vi "Main.vi"(11 "Module Admin":refnum<class "Delacor_lib_QMH_Module Admin.lvclass">) -> ()   [LabVIEW 2020, in "Logging.lvlib"]
doc: "This template is based off of the Queued Message Handler design pattern and the Queued Message Handler project template that ships with LabVIEW.\n\nThe main difference is that the queue is private to this module and communication between modules is performed via Broadcast and Request events.\n\nRequest events are wrapped in public API methods and are handled in the Event Handling Loop (EHL) of this VI. Any module can register for Broadcast events sent by this module. The EHL generates messages based on user interface actions.\n\nThe Message Handling Loop (MHL) processes messages generated by the EHL, or by other messages. The messages are string values, so new messages can be added easily to the Message Cases case structure in the MHL. Each message cluster can also provide an optional value for Message Data, which is a variant that can be converted to whatever message-specific data is required.\n_____\nBased on Delacor QMH Project Template 6.0.0.89."
uses:
  Logging.lvlib
  <vilib>/Delacor/Delacor QMH/Libraries/Module Admin_class/Delacor_lib_QMH_Module Admin.lvclass
  Module Data--cluster.ctl
  <vilib>/Delacor/Delacor QMH/Libraries/Message Queue_class/Delacor_lib_QMH_Message Queue.lvclass/Delacor_lib_QMH_Message Queue.ctl
  Stop Argument--cluster.ctl
  <vilib>/Delacor/Delacor QMH/Libraries/Module Admin_class/Delacor_lib_QMH_Module Admin.lvclass/Delacor_lib_QMH_Module Admin.ctl
  <vilib>/Utility/miscctls.llb/LVPointTypeDef.ctl
  <vilib>/Delacor/Delacor QMH/Libraries/Message Queue_class/Delacor_lib_QMH_Enqueue Message (Single).vi
  <vilib>/Delacor/Delacor QMH/Libraries/Module Admin_class/Delacor_lib_QMH_Get External Launch.vi
  <vilib>/Utility/error.llb/Error Cluster From Error Code.vi
  <vilib>/ErrorRing/Error Ring.xnode
  <vilib>/Delacor/Delacor QMH/Libraries/Message Queue_class/Delacor_lib_QMH_Message Queue.lvclass
  Acquisition/Acquisition.lvlib
  Settings/Settings.lvlib
panel:
  in  "TDMS FILE":bool
  in  "NAME":string
  out "error out":errorcluster
  out "Status":string
  in  "Simulate MHL Error":bool
  in  "Simulate EHL Error":bool
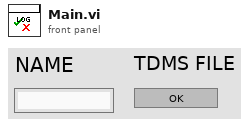
[diagram p1: front panel]
types:
  T1 = typedef "Logging.lvlib/Request Events--cluster.ctl" = cluster{"Stop Module":refnum<user-event>, "Show Panel":refnum<user-event>, "Hide Panel":refnum<user-event>, "Get Module Execution Status":refnum<user-event>, "Show Diagram":refnum<user-event>}
  T2 = typedef "Settings.lvlib/Broadcast Events--cluster.ctl" = cluster{"Module Did Init":refnum<user-event>, "Status Updated":refnum<user-event>, "Error Reported":refnum<user-event>, "Module Did Stop":refnum<user-event>, "Update Module Execution Status":refnum<user-event>, "Task to do":refnum<user-event>, "Nombre task":refnum<user-event>}
  T3 = typedef "Acquisition.lvlib/Broadcast Events--cluster.ctl" = cluster{"Module Did Init":refnum<user-event>, "Status Updated":refnum<user-event>, "Error Reported":refnum<user-event>, "Module Did Stop":refnum<user-event>, "Update Module Execution Status":refnum<user-event>, "Data Analog aquired":refnum<user-event>, "DIGITAL DATA":refnum<user-event>, "TIPO ADQUI":refnum<user-event>}
  T4 = typedef "Logging.lvlib/Module Data--cluster.ctl" = cluster{"Status":string, "ANALOGICO/DIGITAL":bool, "DIGITAL DAQ":bool[], "data":waveform(dbl)[], "NAME":string}
  T5 = enum32{"invalid lock state", "Not Locked", "Locked (No Password)", "Password-protected"}
  T6 = typedef "Logging.lvlib/Stop Argument--cluster.ctl" = cluster{"Origin":string, "Exit via Stop Module Req?":bool, "Wait for Module to stop?":bool}
  T7 = typedef "LVPointTypeDef.ctl" = cluster{"Horizontal":i16, "Vertical":i16}
  T8 = enum32{"Invalid", "Standard", "Closed", "Hidden", "Minimized", "Maximized"}
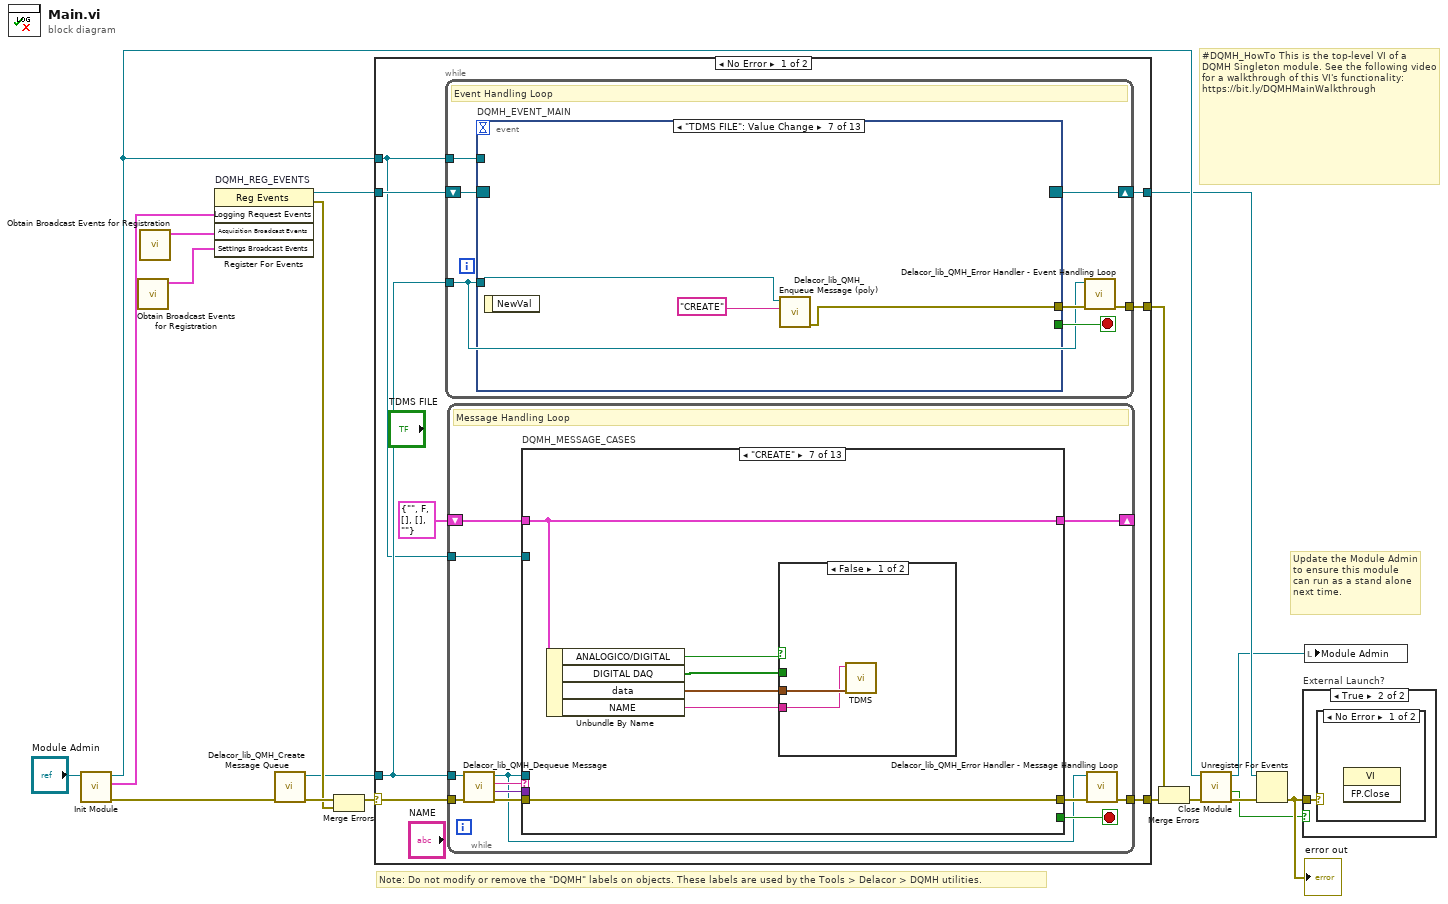
[diagram p0: block diagram]
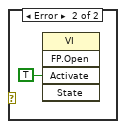
[diagram p3: hidden frame]
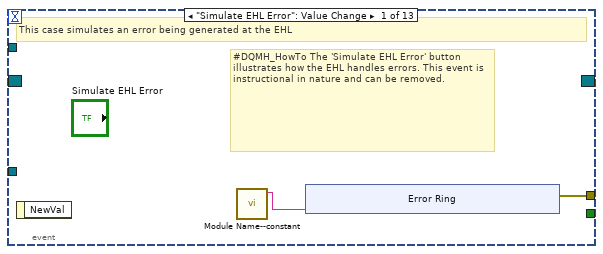
[diagram p4: hidden frame]
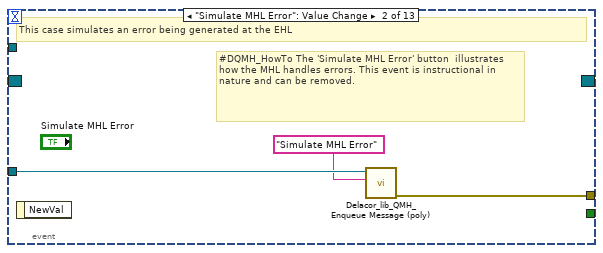
[diagram p5: hidden frame]
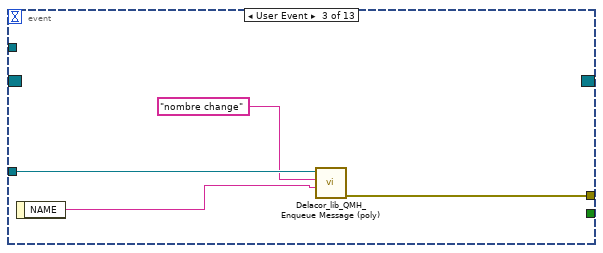
[diagram p6: hidden frame]
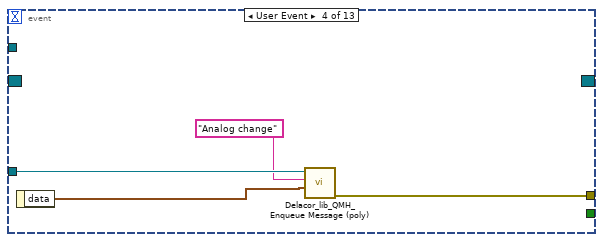
[diagram p7: hidden frame]
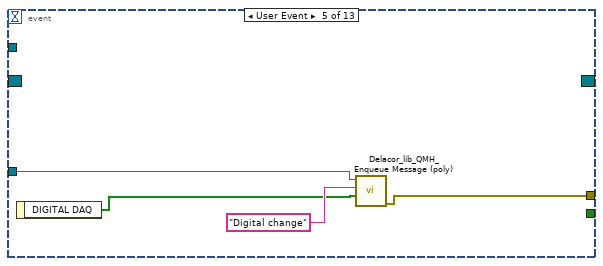
[diagram p8: hidden frame]
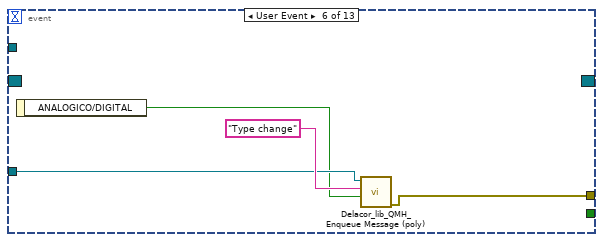
[diagram p9: hidden frame]
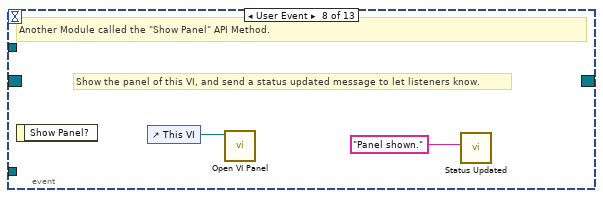
[diagram p10: hidden frame]
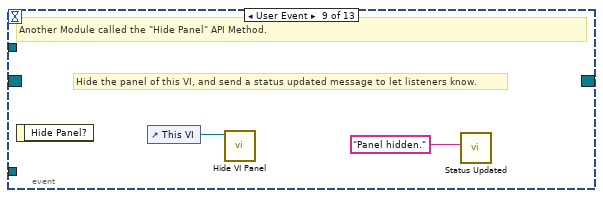
[diagram p11: hidden frame]
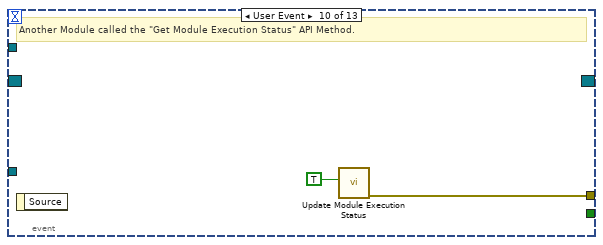
[diagram p12: hidden frame]
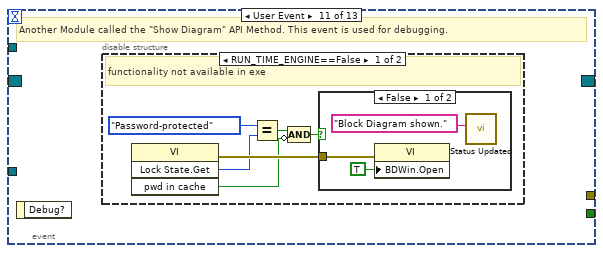
[diagram p13: hidden frame]
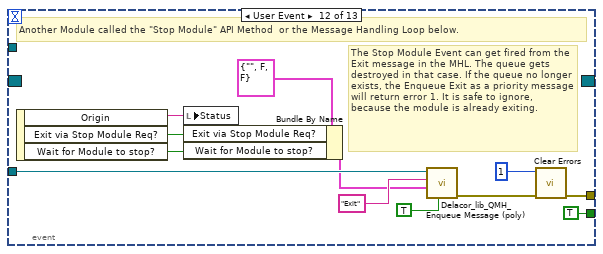
[diagram p16: hidden frame]
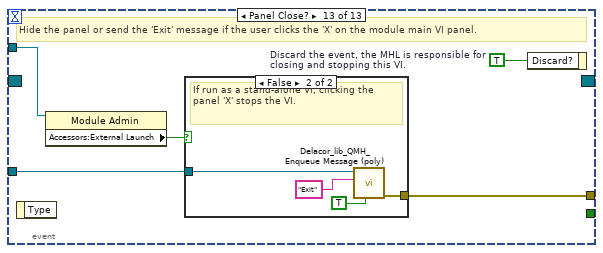
[diagram p17: hidden frame]
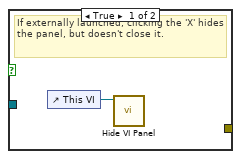
[diagram p18: hidden frame]
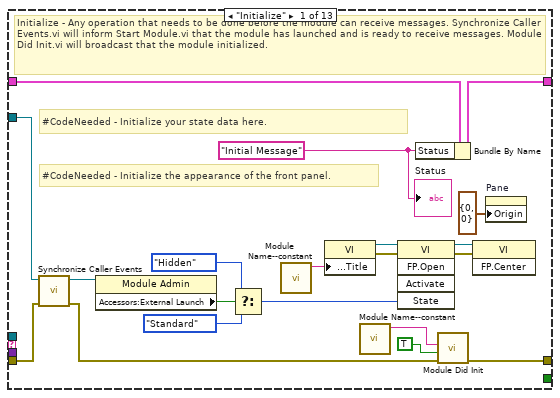
[diagram p19: hidden frame]
diagram:
  # "#DQMH_HowTo This is the top-level VI of a DQMH Singleton module. See the following video for a walkthrough of this VI's functionality: https://bit.ly/DQMHMainWalkthrough"
  # "Note: Do not modify or remove the \"DQMH\" labels on objects. These labels are used by the Tools > Delacor > DQMH utilities."
  # "Update the Module Admin to ensure this module can run as a stand alone next time."
  n1 = call "Init Module.vi"("Singleton Module Admin in"="Module Admin") -> ("error out"=w18:errorcluster, "Logging Request Events"=w7:T1, "Singleton Module Admin out"=w10:refnum<class "Delacor_lib_QMH_Module Admin.lvclass">)  [unwired: 8 in]
  n2 = call "Obtain Broadcast Events for Registration.vi"() -> ("Settings Broadcast Events"=w1:T2)  [unwired: 9 in, 2 out]
  n3 = call "Obtain Broadcast Events for Registration.vi"() -> ("Acquisition Broadcast Events"=w2:T3)  [unwired: 9 in, 2 out]
  n4 = register-events "DQMH_REG_EVENTS"(w7, w2, w1) -> (reference out=w8:refnum<event-registration>, error out=w11:errorcluster)  [unwired: 2 in]
  n5 = call <vilib>:"Delacor_lib_QMH_Create Message Queue.vi"("error in"=w18) -> ("error out"=w13:errorcluster, "Message Queue"=w6:refnum<class "Delacor_lib_QMH_Message Queue.lvclass">)  [unwired: 9 in]
  n6 = Merge Errors(w13, w11) -> (w12:errorcluster)
  n7 = case shown="No Error" w12 {
    selector: w12 -> [w25 w237]
    tunnel: [w27 w236] -> w19
    tunnel: [w24 w242] -> w9
    tunnel: w8 -> [w22 w242]
    tunnel: w6 -> [w21 w235]
    tunnel: [w26 _] -> w16
    tunnel: w10 -> [w20 w238]
    frame No Error {
      n8 = while {
        tunnel: w21 -> [w28]
        shift-right: [w31] -> w24
        shift-left: w22 -> [w32]
        tunnel: [w33] -> w26
        tunnel: w20 -> [w29]
        stop <- w30 stop-if-true
        # "Event Handling Loop"
        n9 = event "DQMH_EVENT_MAIN" shown="[6] \"TDMS FILE\": Value Change" {
          selector: w32 -> [_ _ _ _ _ _ _ _ _ _ _ _ _]
          dyn-events: [_ _ _ _ _ _ _ _ _ _ _ _ _] -> w31
          timeout: _ -> [_ _ _ _ _ _ _ _ _ _ _ _ _]
          tunnel: [_ _ _ _ _ _ _ _ _ _ _ TRUE ("Discard?") _] -> w30
          tunnel: w28 -> [_ w45 w49 w53 w55 w61 w64 _ _ _ _ w88 w95]
          tunnel: [w36 w46 w50 w54 w56 w60 w63 _ _ w71 _ w91 w97] -> w34
          tunnel: w29 -> [_ _ _ _ _ _ _ _ _ _ _ _ w94]
          event "Simulate EHL Error": Value Change {
            # "#DQMH_HowTo The 'Simulate EHL Error' button  illustrates how the EHL handles errors. This event is instructional in nature and can be removed."
            # "This case simulates an error being generated at the EHL"
            n10 = event-data() -> ()  [unwired: 1 in, 1 out]
            n11 = call "Module Name--constant.vi"() -> ("Module Name"=w35:string)  [unwired: 11 in]
            n12 = xnode "Error Ring"("parameter 0"=w35) -> ("error out"=w36:errorcluster)
          }
          event "Simulate MHL Error": Value Change {
            # "#DQMH_HowTo The 'Simulate MHL Error' button  illustrates how the MHL handles errors. This event is instructional in nature and can be removed."
            # "This case simulates an error being generated at the EHL"
            n13 = event-data() -> ()  [unwired: 1 in, 1 out]
            n14 = call-poly <vilib>:"Delacor_lib_QMH_Enqueue Message (poly).vi"("Message"="Simulate MHL Error", "Message Queue in"=w45) -> ("error out"=w46:errorcluster)  [unwired: 8 in, 1 out]
          }
          event User Event {
            n15 = event-data() -> ("NAME"=w48:string)  [unwired: 1 in]
            n16 = call-poly <vilib>:"Delacor_lib_QMH_Enqueue Message (poly).vi"("Message Data"=w48, "Message"="nombre change", "Message Queue in"=w49) -> ("error out"=w50:errorcluster)  [unwired: 7 in, 1 out]
          }
          event User Event {
            n17 = event-data() -> ("data"=w52:waveform(dbl)[])  [unwired: 1 in]
            n18 = call-poly <vilib>:"Delacor_lib_QMH_Enqueue Message (poly).vi"("Message Data"=w52, "Message"="Analog change", "Message Queue in"=w53) -> ("error out"=w54:errorcluster)  [unwired: 7 in, 1 out]
          }
          event User Event {
            n19 = event-data() -> ("DIGITAL DAQ"=w57:bool[])  [unwired: 1 in]
            n20 = call-poly <vilib>:"Delacor_lib_QMH_Enqueue Message (poly).vi"("Message Data"=w57, "Message"="Digital change", "Message Queue in"=w55) -> ("error out"=w56:errorcluster)  [unwired: 7 in, 1 out]
          }
          event User Event {
            n21 = event-data() -> ("ANALOGICO/DIGITAL"=w59:bool)  [unwired: 1 in]
            n22 = call-poly <vilib>:"Delacor_lib_QMH_Enqueue Message (poly).vi"("Message Data"=w59, "Message"="Type change", "Message Queue in"=w61) -> ("error out"=w60:errorcluster)  [unwired: 7 in, 1 out]
          }
          event "TDMS FILE": Value Change {
            n23 = event-data() -> ()  [unwired: 1 in, 1 out]
            n24 = call-poly <vilib>:"Delacor_lib_QMH_Enqueue Message (poly).vi"("Message"="CREATE", "Message Queue in"=w64) -> ("error out"=w63:errorcluster)  [unwired: 8 in, 1 out]
          }
          event User Event {
            # "Show the panel of this VI, and send a status updated message to let listeners know."
            # "Another Module called the \"Show Panel\" API Method."
            n25 = event-data() -> ()  [unwired: 1 in, 1 out]
            n26 = control-ref of="This VI"() -> (w67:refnum<vi>)
            n27 = call "Open VI Panel.vi"("VI"=w67) -> ()  [unwired: 10 in, 1 out]
            n28 = call "Status Updated.vi"("Status"="Panel shown." ("format string")) -> ()  [unwired: 10 in, 1 out]
          }
          event User Event {
            # "Hide the panel of this VI, and send a status updated message to let listeners know."
            # "Another Module called the \"Hide Panel\" API Method."
            n29 = event-data() -> ()  [unwired: 1 in, 1 out]
            n30 = control-ref of="This VI"() -> (w69:refnum<vi>)
            n31 = call "Hide VI Panel.vi"("VI"=w69) -> ()  [unwired: 10 in, 1 out]
            n32 = call "Status Updated.vi"("Status"="Panel hidden." ("format string")) -> ()  [unwired: 10 in, 1 out]
          }
          event User Event {
            # "Another Module called the \"Get Module Execution Status\" API Method."
            n33 = event-data() -> ()  [unwired: 1 in, 1 out]
            n34 = call "Update Module Execution Status.vi"("Running?"=TRUE) -> ("error out"=w71:errorcluster)  [unwired: 10 in]
          }
          event User Event {
            # "Another Module called the \"Show Diagram\" API Method. This event is used for debugging."
            n35 = event-data() -> ()  [unwired: 1 in, 1 out]
            n36 = disable-structure shown="RUN_TIME_ENGINE==False" {
              frame condition #0 (active) {
                # "functionality not available in exe"
                n37 = invoke class="VI" method="Lock State.Get"() -> (error out=w77:errorcluster, "Get Lock State"=w76:T5, "pwd in cache"=w73:bool)  [unwired: 4 in, 1 out]
                n38 = Equal?(x=T5."Password-protected", y=w76) -> (x = y?=w74:bool)
                n39 = Compound Arithmetic op=AND(w74, invert w73) -> (w72:bool)
                n40 = case shown="False" w72 {
                  tunnel: w77 -> [w80 _]
                  frame False {
                    n41 = property class="VI"(error in=w80, "BDWin.Open"=TRUE ("Block Diagram Window:Open")) -> ()  [unwired: 1 in, 2 out]
                    n42 = call "Status Updated.vi"("Status"="Block Diagram shown." ("format string")) -> ()  [unwired: 10 in, 1 out]
                  }
                  frame True {
                    # "Password-protected VI, and the password is not in the cache. Do not show the diagram."
                  }
                }
              }
              frame condition #1 {
              }
            }
          }
          event User Event {
            # "The Stop Module Event can get fired from the Exit message in the MHL. The queue gets destroyed in that case. If the queue no longer exists, the Enqueue Exit as a priority message will return error 1. It is safe to ignore, because the module is already exiting."
            # "Another Module called the \"Stop Module\" API Method  or the Message Handling Loop below."
            n43 = event-data() -> ("Origin"=w87:string, "Exit via Stop Module Req?"=w83:bool, "Wait for Module to stop?"=w82:bool)  [unwired: 1 in]
            n44 = local write "Status"(w87) -> ()
            n45 = Bundle By Name(cluster=T6 {"Origin"="", "Exit via Stop Module Req?"=FALSE, "Wait for Module to stop?"=FALSE} ("Stop Argument"), "Exit via Stop Module Req?"=w83, "Wait for Module to stop?"=w82) -> (w81:T6)
            n46 = call-poly <vilib>:"Delacor_lib_QMH_Enqueue Message (poly).vi"("Priority Message? (F)"=TRUE, "Message Data"=w81, "Message"="Exit", "Message Queue in"=w88) -> ("error out"=w92:errorcluster)  [unwired: 6 in, 1 out]
            n47 = call <vilib>:"Clear Errors.vi"("error in (no error)"=w92, "specific error code to clear (0: all)"=1) -> ("error out"=w91:errorcluster)  [unwired: 4 in, 1 out]
          }
          event Panel Close? {
            w96 = TRUE  # Discard the event, the MHL is responsible for closing and stopping this VI.
            # "Hide the panel or send the 'Exit' message if the user clicks the 'X' on the module main VI panel."
            n48 = event-data() -> ()  [unwired: 1 in, 1 out]
            n49 = property class="Module Admin"(reference=w94) -> ("Accessors:External Launch"=w93:bool)  [unwired: 1 in, 2 out]
            n50 = case shown="False" w93 {
              tunnel: w95 -> [_ w101]
              tunnel: [_ w102] -> w97
              frame True {
                # "If externally launched, clicking the 'X' hides the panel, but doesn't close it."
                n51 = control-ref of="This VI"() -> (w98:refnum<vi>)
                n52 = call "Hide VI Panel.vi"("VI"=w98) -> ()  [unwired: 10 in, 1 out]
              }
              frame False {
                # "If run as a stand-alone VI, clicking the panel 'X' stops the VI."
                n53 = call-poly <vilib>:"Delacor_lib_QMH_Enqueue Message (poly).vi"("Priority Message? (F)"=TRUE, "Message"="Exit", "Message Queue in"=w101) -> ("error out"=w102:errorcluster)  [unwired: 7 in, 1 out]
              }
            }
            n54 = event-data("Discard?"=w96) -> ()  [unwired: 1 in, 1 out]
          }
        }
        n55 = call-dynamic "Delacor_lib_QMH_Error Handler - Event Handling Loop.vi"("error in"=w34, "Message Queue in"=w28) -> ("dup error in"=w33:errorcluster)  [unwired: 8 in, 1 out]
      }
      n56 = while {
        tunnel: w21 -> [w105]
        shift-right: [w109] -> _
        shift-left: T4 {"Status"="", "ANALOGICO/DIGITAL"=FALSE, "DIGITAL DAQ"=[], "data"=[], "NAME"=""} ("Data Cluster") -> [w110]
        tunnel: w25 -> [w113]
        tunnel: [w111] -> w27
        tunnel: w20 -> [w103]
        stop <- w108 stop-if-true
        # "Message Handling Loop"
        n57 = call-dynamic "Delacor_lib_QMH_Dequeue Message.vi"("error in"=w113, "Message Queue in"=w105) -> ("error out"=w112:errorcluster, "Message Data"=w106:variant, "Message"=w107:string, "Message Queue out"=w104:refnum<class "Delacor_lib_QMH_Message Queue.lvclass">)  [unwired: 6 in]
        n58 = case "DQMH_MESSAGE_CASES" shown="\"CREATE\"" w107 {
          selector: w107 -> [_ _ _ _ _ _ _ _ _ _ _ _ w222]
          tunnel: w104 -> [_ _ _ _ _ _ _ _ _ _ w192 w214 _]
          tunnel: w112 -> [w132 w136 w143 w150 w156 w162 w168 w175 w177 w182 w199 w220 w224]
          tunnel: [w130 w136 w142 w149 w156 w162 w168 w174 w177 w181 w195 w217 w225] -> w114
          tunnel: w110 -> [w121 w135 w138 w146 w153 w158 w167 w173 w176 w179 w194 w213 w223]
          tunnel: [w120 w135 w137 w144 w151 w157 w167 w173 w176 w179 w194 w213 w223] -> w109
          tunnel: [_ _ _ _ _ _ _ _ _ _ _ w212 _] -> w108
          tunnel: w106 -> [_ _ w140 w148 w154 w160 _ _ _ _ w193 w211 _]
          tunnel: w103 -> [w122 _ _ _ _ _ _ _ _ _ w191 w206 _]
          frame "Initialize" {
            w116 = "Initial Message" ("Initial Message")
            # "#CodeNeeded - Initialize the appearance of the front panel."
            # "#CodeNeeded - Initialize your state data here."
            # "Initialize - Any operation that needs to be done before the module can receive messages. Synchronize Caller Events.vi will inform Start Module.vi that the module has launched and is ready to receive messages. Module Did Init.vi will broadcast that the module initialized."
            n59 = call "Synchronize Caller Events.vi"("error in (no error)"=w132, "Singleton Module Admin in"=w122) -> ("error out"=w131:errorcluster, "Singleton Module Admin out"=w117:refnum<class "Delacor_lib_QMH_Module Admin.lvclass">)  [unwired: 8 in]
            n60 = property class="Module Admin"(reference=w117) -> ("Accessors:External Launch"=w126:bool)  [unwired: 1 in, 2 out]
            n61 = Select(t=T8."Hidden" ("State"), s=w126, f=T8."Standard" ("State")) -> (s? t:f=w123:T8)
            n62 = call "Module Name--constant.vi"() -> ("Module Name"=w129:string)  [unwired: 11 in]
            n63 = property class="VI"("Front Panel.Title"=w129) -> (reference out=w128:refnum<vi>, error out=w134:errorcluster)  [unwired: 2 in]
            n64 = call "Module Name--constant.vi"() -> ("Module Name"=w118:string)  [unwired: 11 in]
            n65 = invoke class="VI" method="FP.Open"(reference=w128, error in=w134, "State"=w123) -> (reference out=w127:refnum<vi>, error out=w133:errorcluster)  [unwired: 2 in, 3 out]
            n66 = Bundle By Name(cluster=w121, "Status"=w116) -> (w120:T4)
            n67 = call "Module Did Init.vi"("error in (no error)"=w131, "Initialized?"=TRUE, "Origin"=w118) -> ("error out"=w130:errorcluster)  [unwired: 8 in]
            n68 = invoke class="VI" method="FP.Center"(reference=w127, error in=w133) -> ()  [unwired: 1 in, 3 out]
            n69 = property on="Pane" class="Pane"("Origin"=T7 {"Horizontal"=0, "Vertical"=0}) -> ()  [unwired: 2 in, 2 out]
            "Status" <- w116
          }
          frame "---Module Specific---" {
            # "Separator -- The following cases handle messages specific to this Module."
          }
          frame "nombre change" {
            n70 = Variant To Data(error in=w143, type="", Variant=w140) -> (data=w139:string, error out=w142:errorcluster)
            n71 = Bundle By Name(cluster=w138, "NAME"=w139) -> (w137:T4)
          }
          frame "Analog change" {
            n72 = Variant To Data(error in=w150, type=waveform(dbl)[] [] ("data"), Variant=w148) -> (data=w147:waveform(dbl)[], error out=w149:errorcluster)
            n73 = Bundle By Name(cluster=w146, "data"=w147) -> (w144:T4)
          }
          frame "Digital change" {
            n74 = Variant To Data(type=bool[] [] ("DIGITAL DAQ"), Variant=w154) -> (data=w155:bool[])  [unwired: 1 in, 1 out]
            n75 = Bundle By Name(cluster=w153, "DIGITAL DAQ"=w155) -> (w151:T4)
          }
          frame "Type change" {
            n76 = Variant To Data(type=FALSE ("ANALOGICO/DIGITAL"), Variant=w160) -> (data=w161:bool)  [unwired: 1 in, 1 out]
            n77 = Bundle By Name(cluster=w158, "ANALOGICO/DIGITAL"=w161) -> (w157:T4)
          }
          frame "CREATE" {
            n78 = Unbundle By Name(w167) -> ("ANALOGICO/DIGITAL"=w166:bool, "DIGITAL DAQ"=w165:bool[], "data"=w164:waveform(dbl)[], "NAME"=w163:string)
            n79 = case shown="False" w166 {
              tunnel: w165 -> [_ w171]
              tunnel: w164 -> [w170 _]
              tunnel: w163 -> [w169 w172]
              frame False {
                n80 = call "TDMS.vi"("ANALOGICO"=w170, "group name in (Untitled)"=w169) -> ()  [unwired: 10 in]
              }
              frame True {
                n81 = call "DIGITAL TDMS.vi"("DIGITAL DAQ 2"=w171, "NAME"=w172) -> ()  [unwired: 10 in]
              }
            }
          }
          frame "---Copy This Frame---" {
            # "Duplicate this frame when creating new messages.  Change this comment in the duplicated frame to describe this message."
            n82 = Merge Errors(w175) -> (w174:errorcluster)
          }
          frame "---Exit and Error Handling---" {
            # "Separator - The following cases handle errors and exit messages."
          }
          frame "Simulate MHL Error" {
            # "#DQMH_HowTo The 'Simulate MHL Error' button  illustrates how the MHL handles errors. This event is instructional in nature and can be removed."
            # "Simulate an error occurring at the MHL"
            n83 = call "Module Name--constant.vi"() -> ("Module Name"=w178:string)  [unwired: 11 in]
            n84 = xnode "Error Ring"("parameter 0"=w178) -> ("error out"=w180:errorcluster)
            n85 = Merge Errors(w182, w180) -> (w181:errorcluster)
          }
          frame "Error" {
            # "#CodeRecommended - If you ever change the name of this \"Error\" message, you'll need to update the name in the Check Loop Error.vi as well."
            # "#CodeRecommended - If the module is running in standalone mode (External Launch = FALSE), this code will pop up an error dialog and call the 'Exit' message if an error occurs. Add more fine-grained error handling here."
            # "Error - Check the error message data and respond accordingly. This message is sent by the \"Error Handler\" VIs at the end of each loop in this application."
            n86 = property class="Module Admin"(reference=w191) -> ("Accessors:External Launch"=w190:bool)  [unwired: 1 in, 2 out]
            n87 = Variant To Data(error in=w199, type=errorcluster {"status"=FALSE, "code"=0, "source"=""} ("error constant"), Variant=w193) -> (data=w200:errorcluster, error out=w197:errorcluster)
            n88 = call "Error Reported.vi"("Error"=w200) -> ()  [unwired: 10 in, 1 out]
            n89 = case shown="False" w190 {
              tunnel: [w205 _] -> w196
              tunnel: w192 -> [w203 _]
              tunnel: w200 -> [w204 _]
              frame False {
                # "If the module is running standalone, then pop up an error dialog and call the \"Exit\" message."
                n90 = call <vilib>:"Simple Error Handler.vi"("error in (no error)"=w204) -> ()  [unwired: 4 in, 5 out]
                n91 = call-poly <vilib>:"Delacor_lib_QMH_Enqueue Message (poly).vi"("Priority Message? (F)"=TRUE, "Message"="Exit", "Message Queue in"=w203) -> ("error out"=w205:errorcluster)  [unwired: 7 in, 1 out]
              }
              frame True {
                # "If the module was launched externally, calling the Error Reported broadcast VI is the only action performed by the \"Error\" message. The module's caller can then process the error appropriately."
              }
            }
            n92 = Merge Errors(w197, w196) -> (w195:errorcluster)
            n93 = local write "error out"(w195) -> ()
          }
          frame "Exit" {
            w210 = 91  # 91: not all Exit messages will have an argument
            w212 = TRUE  # Stop the VI
            # "Release the message queue reference"
            # "#CodeNeeded - Add any required cleanup code here"
            # "Exit - Exit the application."
            n94 = Variant To Data(error in=w220, type=T6 {"Origin"="", "Exit via Stop Module Req?"=FALSE, "Wait for Module to stop?"=FALSE} ("Stop Argument"), Variant=w211) -> (data=w208:T6, error out=w216:errorcluster)
            n95 = call <vilib>:"Clear Errors.vi"("error in (no error)"=w216, "specific error code to clear (0: all)"=w210) -> ("error out"=w219:errorcluster)  [unwired: 4 in, 1 out]
            n96 = control-ref of="This VI"() -> (w207:refnum<vi>)
            n97 = call-dynamic "Delacor_lib_QMH_Release Message Queue.vi"("error in"=w219, "Message Queue"=w214) -> ("error out"=w218:errorcluster)  [unwired: 9 in]
            n98 = call "Handle Exit.vi"("Stop Argument"=w208, "Admin in"=w206, "VI reference"=w207) -> ("error out"=w215:errorcluster)  [unwired: 7 in, 1 out]
            n99 = Merge Errors(w218, w215) -> (w217:errorcluster)
          }
          frame Default {
            # "'Default' case only runs if there is a message that isn't defined in any of the other cases.  Output a programming error."
            n100 = call "Module Name--constant.vi"() -> ("Module Name"=w221:string)  [unwired: 11 in]
            n101 = xnode "Error Ring"("parameter 0"=w222, "parameter 1"=w221) -> ("error out"=w226:errorcluster)
            n102 = Merge Errors(w224, w226) -> (w225:errorcluster)
          }
        }
        n103 = call-dynamic "Delacor_lib_QMH_Error Handler - Message Handling Loop.vi"("error in"=w114, "Message Queue in"=w104) -> ("dup error in"=w111:errorcluster)  [unwired: 8 in, 1 out]
      }
    }
    frame Error {
      # "Synchronize Caller Events.vi will inform Start Module.vi that the module has launched and will let the code calling Start Module.vi register for broadcasts and would permit the caller receive the broadcast that an error occurred at launch time."
      n104 = call-dynamic "Delacor_lib_QMH_Release Message Queue.vi"("error in"=w237, "Message Queue"=w235) -> ("error out"=w236:errorcluster)  [unwired: 9 in]
      n105 = call "Synchronize Caller Events.vi"("Singleton Module Admin in"=w238) -> ("error out"=w243:errorcluster)  [unwired: 9 in, 1 out]
      n106 = call "Module Name--constant.vi"() -> ("Module Name"=w241:string)  [unwired: 11 in]
      n107 = Format Into String(format string="An error occurred during initialization. %s is no longer running.", w241) -> (resulting string=w239:string)  [unwired: 2 in, 1 out]
      n108 = Merge Errors(w236, w243) -> (w244:errorcluster)
      n109 = call "Error Reported.vi"("Additional Information"=w239, "Error"=w244) -> ()  [unwired: 9 in, 1 out]
    }
  }
  n110 = Merge Errors(w16, w19) -> (w15:errorcluster)
  n111 = call "Close Module.vi"("error in (no error)"=w15, "Module Admin in"=w10) -> ("error out"=w17:errorcluster, "External Launch"=w3:bool, "Module Admin out"=w4:refnum<class "Delacor_lib_QMH_Module Admin.lvclass">)  [unwired: 7 in]
  n112 = Unregister For Events(event registration refnum=w9, error in=w17) -> (error out=w14:errorcluster)
  "error out" <- w14
  n113 = case "External Launch?" shown="True" w3 {
    tunnel: w14 -> [_ w245]
    frame False {
    }
    frame True {
      n114 = case shown="No Error" w245 {
        frame No Error {
          n115 = invoke class="VI" method="FP.Close"() -> ()  [unwired: 3 in, 3 out]
        }
        frame Error {
          n116 = invoke class="VI" method="FP.Open"("Activate"=TRUE ("Activate?")) -> ()  [unwired: 4 in, 5 out]
        }
      }
    }
  }
  n117 = local write "Module Admin"(w4) -> ()
